vi "Convert and Scale.vi"(3 "Number In":u16, 4 "Scale Value":dbl) -> (5 "Converter Number Out":dbl)   [LabVIEW 2014]
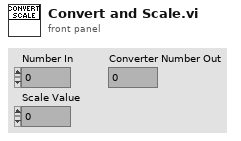
[diagram p1: front panel]
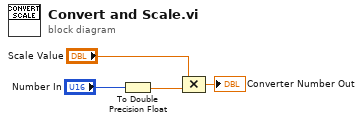
[diagram p0: block diagram]
diagram:
  n1 = To Double Precision Float(number="Number In") -> (double precision float=w3:dbl)
  n2 = Compound Arithmetic op=MULTIPLY("Scale Value", w3) -> (→"Converter Number Out":dbl)
